vi "THz Time(SR830_ESP300)_Delay_LGS.vi"(1 "ESP300 Axis1":i8=1, 2 "ESP300 Address1":string="1", 4 "Lockin Address":string="12") -> ()   [LabVIEW 2010]
uses:
  <vilib>/Utility/file.llb/Write To Spreadsheet File (DBL).vi
panel:
  out "Boolean 2":bool
  in  "Position 3":sgl=3.0 format="%#.4f"
  in  "Set Position 2":bool
  out "error out":errorcluster
  out "Position 2":dbl[](array[numeric])=[3.0] format="%.6f"
  in  "error in":errorcluster
  out "Running":bool caption="Mercury_GCS_Configuration_Setup.vi is running"
  out "Conn. Axis":string[](array[string])=["1"]
  out "Identification":string="(c)2013 Physik Instrumente(PI) Karlsruhe, C-863.11,0,1.3.0.7"
  in  "SaveFile name":string="t"
  in  "Interdelay (ms)":dbl=10.0
  in  "pre delay(ms)":dbl=100.0
  out "Current deceleration":dbl=100.0
  in  "Acceleration":dbl
  out "Current acceleration":dbl=100.0
  in  "Set Acc":bool
  out "Current Velocity":dbl=25.0
  in  "Delay1 Stage":dbl
  in  "Set Velocity":bool
  in  "Reset Range":bool
  out "Boolean":bool
  out "MinValue":dbl format="%#.3p"
  out "MinPosition":dbl format="%#.3f"
  out "Lock-in Y-Channel":dbl=-8.0036e-11 format="%#.3p"
  out "Lock-in X-Channel":dbl=5.62071e-10 format="%#.3p"
  out "THz Time-domain Signal Wave":cluster{"x-axis":sgl[], "y-axis":dbl[]}(graph)={"x-axis"=[-2.75, -2.745, -2.74, -2.735, -2.73, -2.725, -2.72, -2.715, -2.71, -2.705, -2.7, -2.695, -2.69, -2.685, -2.68, -2.675, -2.67, -2.665, -2.66, -2.655, -2.65, -2.645, -2.64, -2.635, -2.63, -2.625, -2.62, -2.615, -2.61, -2.605, -2.6, -2.595, -2.59, -2.585, -2.58, -2.575, -2.57, -2.565, -2.56, -2.555, -2.55, -2.545, -2.54, -2.535, -2.53, -2.525, -2.52, -2.515, -2.51, -2.505, -2.5, -2.4950001, -2.49, -2.485, -2.48, -2.475, -2.47, -2.465, -2.46, -2.455, -2.45, -2.445, -2.44, -2.435, -2.43, -2.425, -2.42, -2.415, -2.41, -2.405, -2.4, -2.395, -2.39, -2.385, -2.38, -2.375, -2.3700001, -2.365, -2.36, -2.355, -2.35, -2.345, -2.34, -2.335, -2.33, -2.325, -2.32, -2.315, -2.31, -2.305, -2.3, -2.295, -2.29, -2.285, -2.28, -2.275, -2.27, -2.265, -2.26, -2.255, -2.25, -2.2450001, -2.24, -2.235, -2.23, -2.225, -2.22, -2.215, -2.21, -2.205, -2.2, -2.195, -2.19, -2.185, -2.18, -2.175, -2.17, -2.165, -2.16, -2.155, -2.15, -2.145, -2.14, -2.135, -2.13, -2.125, -2.1200001, -2.115, -2.1100001, -2.105, -2.1, -2.095, -2.09, -2.085, -2.08, -2.075, -2.07, -2.065, -2.06, -2.055, -2.05, -2.045, -2.04, -2.035, -2.03, -2.025, -2.02, -2.015, -2.01, -2.005, -2.0, -1.995, -1.99, -1.985, -1.98, -1.975, -1.97, -1.965, -1.96, -1.955, -1.95, -1.945, -1.94, -1.9350001, -1.9300001, -1.9250001, -1.9200001, -1.915, -1.91, -1.905, -1.9, -1.895, -1.89, -1.885, -1.88, -1.875, -1.87, -1.865, -1.86, -1.855, -1.85, -1.845, -1.84, -1.835, -1.83, -1.825, -1.82, -1.815, -1.8100001, -1.8050001, -1.8000001, -1.7950001, -1.79, -1.785, -1.78, -1.775, -1.77, -1.765, -1.76, -1.755, -1.75, -1.745], "y-axis"=array[202 elements]}
  in  "Autosave Directory for Long-term Average Scan":path=path "D:/Soon/140901_delay_test/2_VC_delay_ESP_-2.35/2_ESP_delay"
  out "Phase":cluster{"f0":dbl, "df":dbl, "magnitude":dbl[]}(graph)={"f0"=0.0, "df"=0.14851486070616432, "magnitude"=[3.141592653589793, -1.135986580040852, 2.1022109002271616, -0.606224595657138, 2.920681076611292, 0.21556372083252148, -2.5451476520052716, 0.9923939961615453, -1.7463610341623916, 1.8333042754436455, -0.8359836995409918, 2.75507186449797, 0.09169493821671801, -2.671398777194605, 0.9252867844951119, -1.8804339733205764, 1.635385337194291, -1.1519546083083008, 2.397714684588004, 1.2104854849686713, -2.8637531980944555, 1.949308293908791, 0.7861851325694362, 2.05817428941482, -0.20905665475156449, 2.1403175698295978, 0.5803199632569114, 2.0240075732653433, 2.7198480916992196, 1.4424734657875855, -2.685986408674916, 1.659408491765386, -1.770724027329074, 2.081076418078137, 0.08608209088206076, 2.493628967277787, 1.3416383131006835, 2.776511176774577, 1.7385392296843876, 2.910643788155704, 2.0733616555355256, 2.1476846304355526, 2.3752410087260474, 1.8644630479941513, 2.5623127875118348, 2.148045822962683, 2.289396670128229, 2.4297700200498875, 2.095071647481632, 2.572627457331977, 2.109964594823839, 2.6198261810673187, 2.2914243248471258, 2.3594402988625824, 2.5589534913230425, 1.7745700362271504, 2.954962782799749, 1.86194698187105, -3.1249566392866623, 2.2303719482942626, 2.6892266936683993, 2.5935042746540447, 2.41043968808954, 2.6541419887600273, 2.683074815417406, 2.1668243385246915, -3.070776678111956, 2.2892022436016632, -2.135166602508625, 2.7313396286767393, 1.2942375262133383, -2.98549486935882, 2.211769682179136, -1.9765629636412416, 2.8315046162560114, 0.8982661941803926, 3.0979638891430006, 1.3338431160230941, 2.9572589462558923, 0.4208158598849399, -3.084879211462056, 1.1546365000649987, -2.426896356838734, 2.1224318208935746, -1.0822400276671367, -3.138191445873515, 1.3677675484659175, -2.1384004116313586, 2.2666526927596524, -0.9626777899091671, 2.9711856946896824, 0.5728247348162799, -2.816675001259512, 1.473325365303859, -2.6794056673427953, 1.5349065678241745, -2.6858532380239843, 1.534598210049353, -2.4469347300537185, 2.0442041388150147, -2.311182814513963]}
  out "elapsed time":string=" 0 h  16 m  48 s"
  in  "OK Button":bool
  out "Data Type":string="outp ? 1"
  in  "Enum":enum16{"X", "Y", "Abs"}(ring)
  out "MaxValue":dbl format="%#.3p"
  out "MaxPosition":dbl format="%#.3f"
  in  "Position":sgl format="%#.4f"
  in  "Find Max":bool
  in  "Set Position":bool
  in  "Save Data":bool
  in  "SCAN":bool
  in  "Exit Program":bool
  out "Amplitude":cluster{"f0":dbl, "df":dbl, "magnitude":dbl[]}(graph)={"f0"=0.0, "df"=0.14851486070616432, "magnitude"=[2.6915991854888386e-11, 8.375656748039542e-10, 2.235834721082622e-09, 3.4157684600132285e-09, 4.2435755658762315e-09, 4.472539329076285e-09, 4.2347337941880014e-09, 3.6229569047721997e-09, 2.7975925998611847e-09, 2.0909687588148054e-09, 1.4776684583256283e-09, 1.0684148893892852e-09, 7.434640997068466e-10, 5.034295148742816e-10, 3.3364314234066716e-10, 1.9577697939408548e-10, 1.2523927442263667e-10, 4.429210924914903e-11, 2.573647079693204e-11, 1.4182414959459453e-11, 2.7755861329404263e-12, 1.4087176698727024e-11, 1.3906256401648906e-12, 1.3855617151926235e-11, 2.3183905698719347e-12, 1.3260260840826552e-11, 1.6764421372823549e-12, 9.240136905598061e-12, 4.112473401393782e-12, 9.698672089635608e-12, 6.399880474780534e-12, 1.3297238354970657e-11, 4.270910531055341e-12, 1.194277964154244e-11, 2.0143741595524134e-12, 8.19663059000381e-12, 4.499163612930761e-12, 4.984976956409621e-12, 5.930135725317639e-12, 2.6529048225466805e-12, 6.413329122555876e-12, 1.5875211615976485e-12, 5.603892306521492e-12, 3.0822718239556447e-12, 3.773490804705028e-12, 4.266071720358043e-12, 2.7269286375688967e-12, 4.04702550108293e-12, 3.1385561228088536e-12, 3.5820473163129804e-12, 3.4584571573909894e-12, 2.8260585036815302e-12, 3.954420907012932e-12, 2.109422403518565e-12, 4.405123782627864e-12, 2.328141166049999e-12, 4.110618048699576e-12, 3.7699178777659875e-12, 2.75243386150393e-12, 4.1423186986189514e-12, 1.889383468271808e-12, 3.468042829240754e-12, 2.7069840219363736e-12, 2.355134561389352e-12, 3.3764264273860032e-12, 2.5890110570824253e-12, 2.645733242043269e-12, 4.509912096670506e-12, 7.24673781011345e-13, 5.531658054842724e-12, 1.7743067719520671e-12, 3.936201982796357e-12, 4.271899404256137e-12, 8.217749918070464e-13, 5.699197262594634e-12, 1.5430271083565579e-12, 5.25759708946632e-12, 1.449496509764676e-12, 5.3347687277906044e-12, 1.804360465622194e-12, 6.9752988572067005e-12, 4.2197168647319695e-12, 5.704160353607782e-12, 5.79769144265315e-12, 2.0168312984405185e-12, 6.483488385921406e-12, 4.16443233788095e-12, 5.524003351010582e-12, 6.9219189903466406e-12, 3.2560936701576393e-12, 7.2038923234186815e-12, 2.643003207182121e-12, 6.1557127448571425e-12, 3.009475442598e-12, 5.064751562703159e-12, 2.590926363995777e-12, 5.492940598962602e-12, 3.266879593571407e-12, 5.207284837307166e-12, 3.5754755911677846e-12, 2.6128905192061403e-12]}
  in  "Short term \nAverage#":i8=2
  out "Numeric 2":i8=15
  in  "Long term Average#":i8=16
  in  "Step":sgl=0.005 min=0 max=10000 format="%.3f"
  in  "End Postion":sgl=-1.75 min=-400 max=400 format="%#.3f"
  in  "Start Position":sgl=-2.75 min=-400 max=400 format="%#.3f"
  # "This Program Run First (1) and then Run the Approach Program (2)"
  # "THz Experiment"
  # "``"
  # "Auto-offset"
  # "Input Data"
  # "Delay Line (ESP300)"
  # "Point Avg"
  # "Long Avg"
  # "Turn Number"
  # "mm"
  # "mm"
  # "MAX"
  # "MIN"
  # "other step\nposition"
  # "stage \nposition"
  # "stage \nposition"
  # "value"
  # "value"
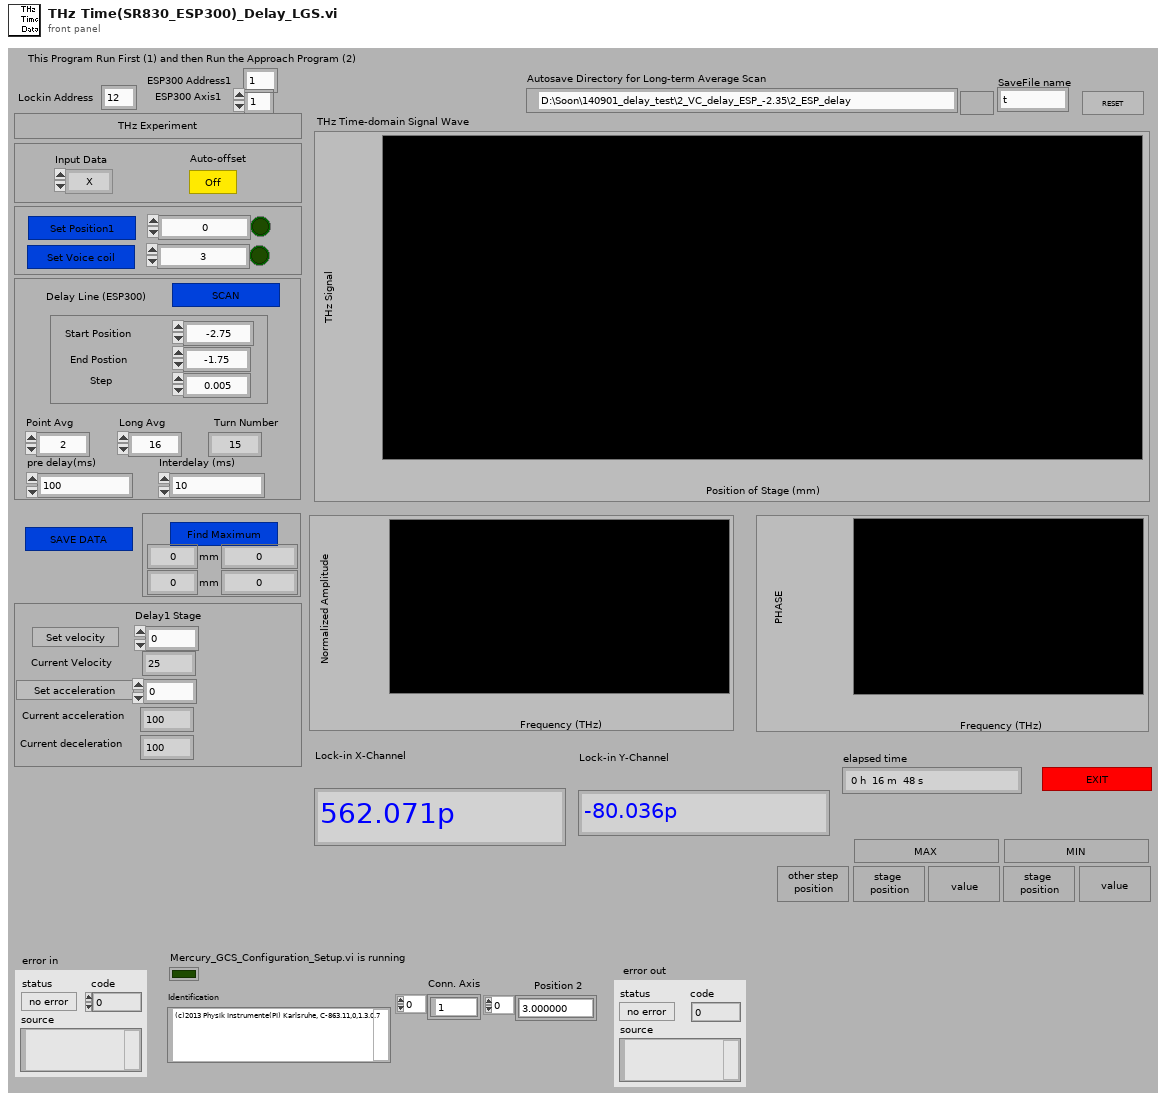
[diagram p1: front panel]
types:
  T1 = cluster{"System no.":i32, "error out":errorcluster}
  T2 = cluster{"Step Number":i32, "Step":sgl, "Start Position":sgl, "Time-out":i32, "Lockin Address":string, "Short term \nAverage#":i8, i32, "ESP300 Axis1":i8, "Value":string, "pre delay(ms)":dbl, "Interdelay (ms)":dbl, "Autosave Directory for Long-term Average Scan":path}
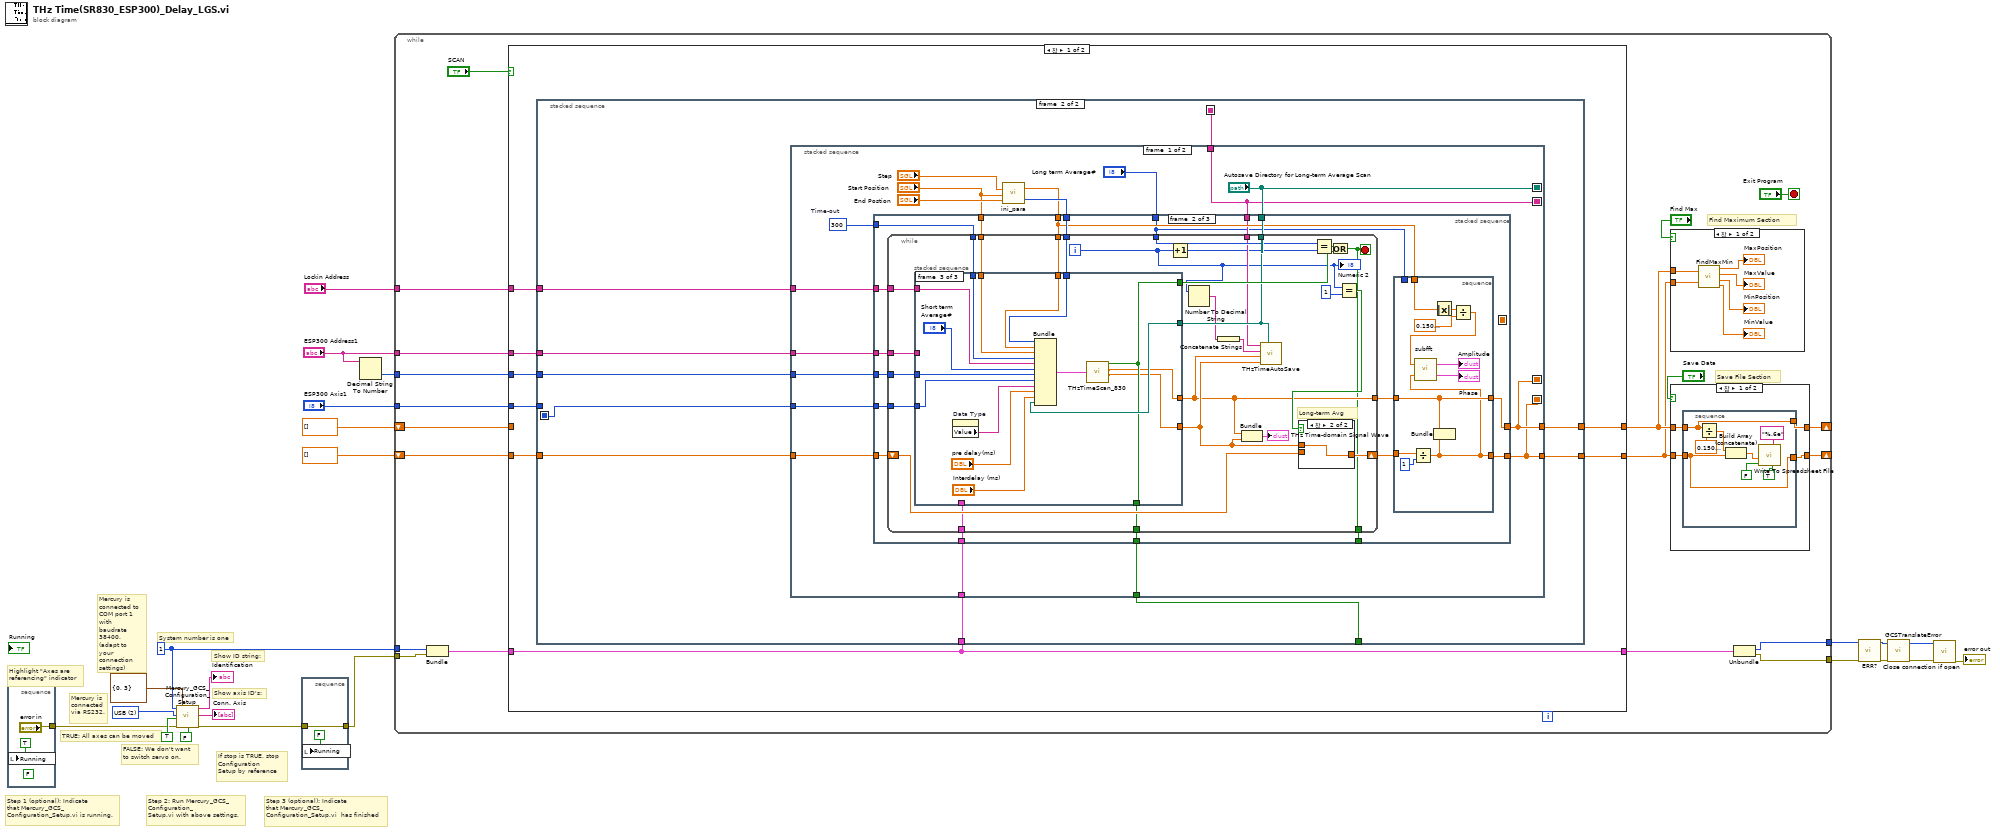
[diagram p0: block diagram]
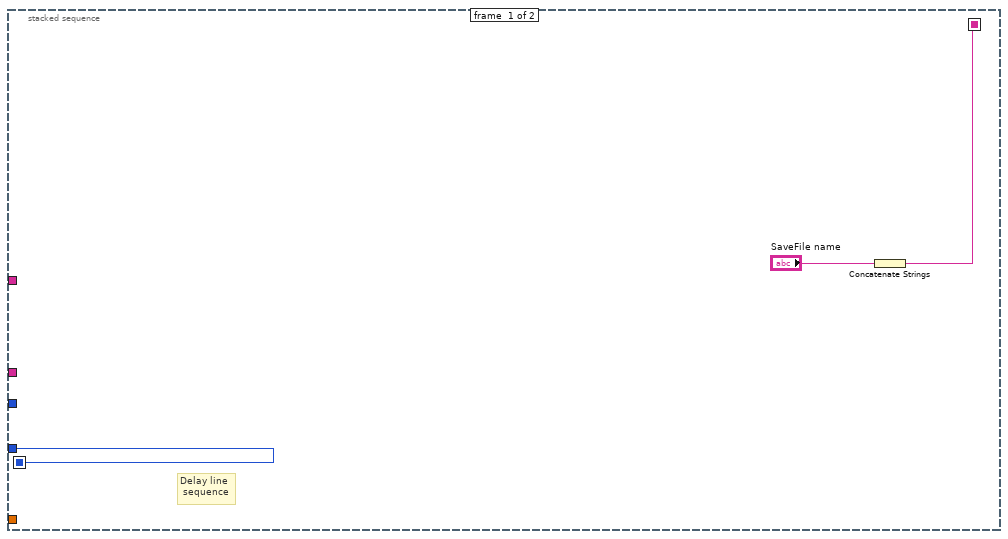
[diagram p4: hidden frame]
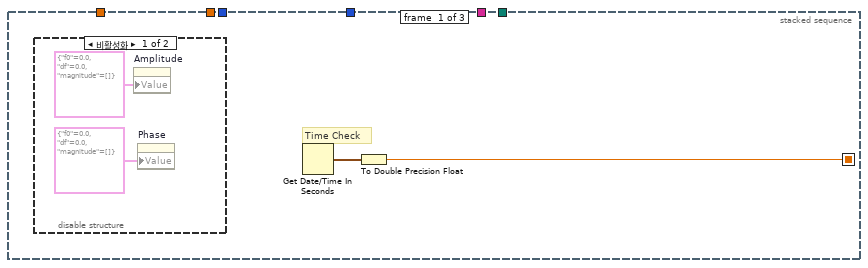
[diagram p5: hidden frame]
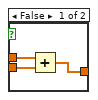
[diagram p7: hidden frame]
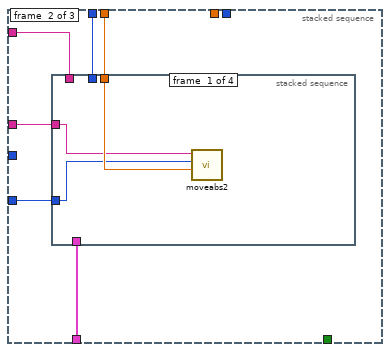
[diagram p9: hidden frame]
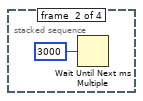
[diagram p10: hidden frame]
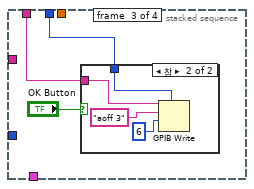
[diagram p11: hidden frame]
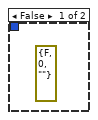
[diagram p12: hidden frame]
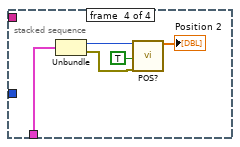
[diagram p13: hidden frame]
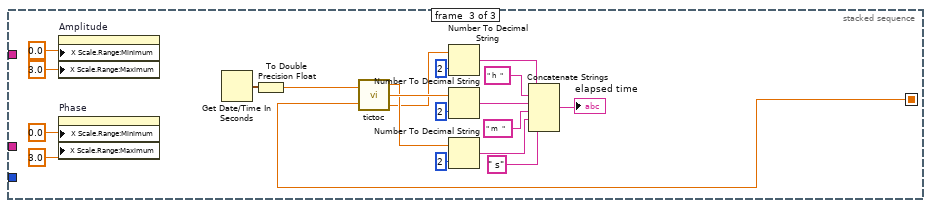
[diagram p14: hidden frame]
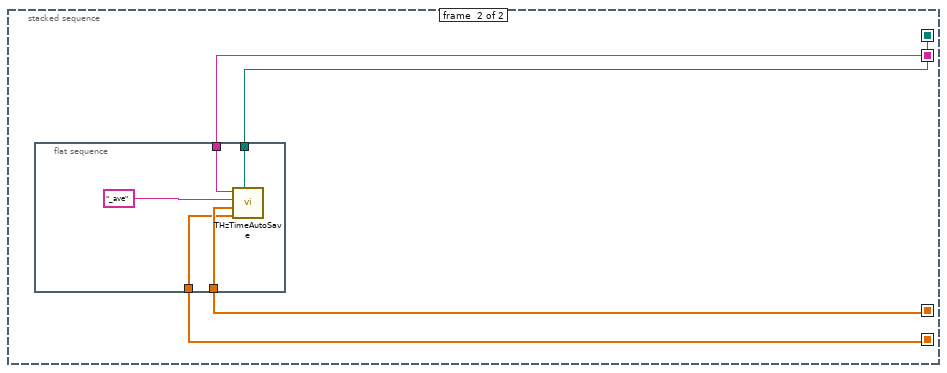
[diagram p15: hidden frame]
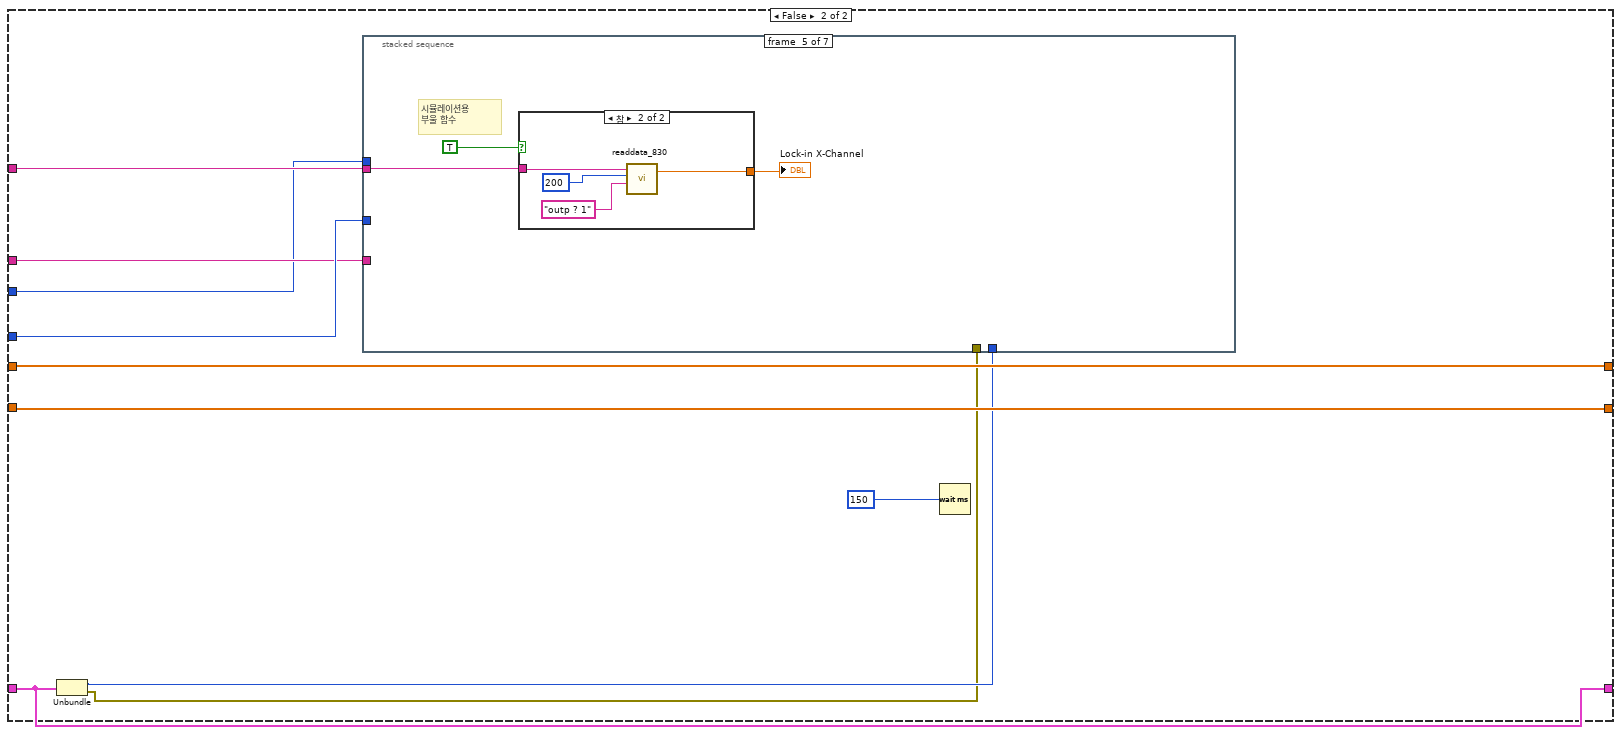
[diagram p16: hidden frame]
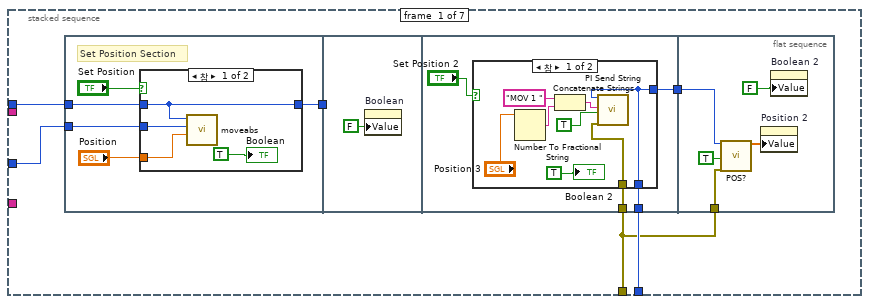
[diagram p17: hidden frame]
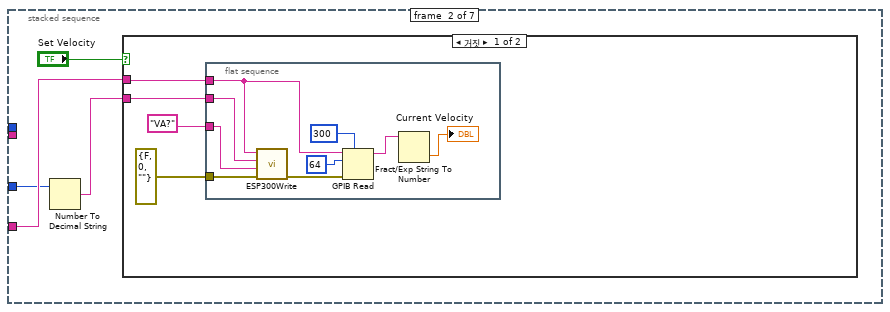
[diagram p20: hidden frame]
diagram:
  w8 = u16 2 items=["RS232", "RS232 DaisyChain", "USB", "USB_DaisyChain"] ("Interface")
  w7 = 1 ("System no.")
  # "Mercury is\nconnected\nvia RS232."
  # "If stop is TRUE, stop \nConfiguration\nSetup by reference"
  # "Mercury is\nconnected to\nCOM port 1\nwith baudrate\n38400.\n(adapt to your\nconnection\nsettings)"
  # "Step 3 (optional): Indicate\nthat Mercury_GCS_\nConfiguration_Setup.vi  has finished"
  # "Step 2: Run Mercury_GCS_\nConfiguration_\nSetup.vi with above settings."
  # "Step 1 (optional): Indicate\nthat Mercury_GCS_\nConfiguration_Setup.vi is running."
  # "Highlight \"Axes are\nreferencing\" indicator"
  # "Show axis ID's:"
  # "Show ID string:"
  # "FALSE: We don't want\nto switch servo on."
  # "TRUE: All axes can be moved"
  # "System number is one"
  n1 = stacked-sequence {
    tunnel: ["error in"] -> w11
    frame #0 {
      (unwired) FALSE ("stop")
      n2 = local write "Running"(TRUE ("Running")) -> ()
    }
  }
  n3 = call "Mercury_GCS_Configuration_Setup.vi"("System no."=w7, "Interface"=w8, "All axes?"=TRUE, "error in"=w11, "RS232 settings"=cluster{"RS232 Portnumber":i32, "Baudrate":u16} {"RS232 Portnumber"=0, "Baudrate"=3}, "Switch servo on?"=FALSE ("Use dialog to define\nconnected stages?")) -> ("Identification"=→"Identification":string, "Conn. \nAxes"=→"Conn. Axis":string[], "error out"=w12:errorcluster)  [unwired: 7 in, 4 out]
  n4 = stacked-sequence {
    tunnel: w12 -> [w25]
    tunnel: [w25] -> w6
    frame #0 {
      n5 = local write "Running"(FALSE ("Running")) -> ()
    }
  }
  n6 = Decimal String To Number(string="ESP300 Address1") -> (number=w16:i32)  [unwired: 2 in, 1 out]
  n7 = while {
    tunnel: "ESP300 Axis1" -> [w41]
    tunnel: "Lockin Address" -> [w33]
    shift-right: [w38] -> _
    shift-left: sgl[] [] -> [w40]
    shift-right: [w37] -> _
    shift-left: dbl[] [] -> [w39]
    tunnel: "ESP300 Address1" -> [w34]
    tunnel: w16 -> [w32]
    tunnel: w7 -> [w31]
    tunnel: w6 -> [w30]
    tunnel: [w27] -> w2
    tunnel: [w26] -> w1
    stop <- "Exit Program" stop-if-true
    # "Save File Section"
    # "Find Maximum Section"
    n8 = Bundle("System no."=w31, "error out"=w30) -> (w29:T1)  [unwired: 1 in]
    n9 = case shown="참" "SCAN" {
      tunnel: w41 -> [w73 w245]
      tunnel: [w72 w242] -> w36
      tunnel: [w71 w241] -> w35
      tunnel: w40 -> [_ w242]
      tunnel: w39 -> [w70 w241]
      tunnel: w34 -> [w69 w243]
      tunnel: w33 -> [w68 w240]
      tunnel: w32 -> [w67 w239]
      tunnel: w29 -> [w66 w236]
      tunnel: [w66 w236] -> w28
      frame True {
        n10 = stacked-sequence {
          seq-local: [w76 _] -> [_ w79]
          seq-local: [w74 _] -> [_ w80]
          tunnel: w73 -> [w76 _]
          tunnel: [_ w86] -> w72
          tunnel: [_ w85] -> w71
          tunnel: w70 -> [_ w84]
          tunnel: w69 -> [_ w83]
          tunnel: w68 -> [_ w82]
          tunnel: w67 -> [_ w81]
          tunnel: [_ w77] -> _
          tunnel: w66 -> [_ w78]
          frame #0 {
            # "Delay line\n sequence"
            n11 = Concatenate Strings("SaveFile name") -> (w74:string)
          }
          frame #1 {
            n12 = stacked-sequence {
              seq-local: [w94 _] -> [_ w228]
              seq-local: [w93 _] -> [_ w227]
              seq-local: ["Autosave Directory for Long-term Average Scan" _] -> [_ w229]
              seq-local: [w89 _] -> [_ w230]
              tunnel: w79 -> [w104 _]
              tunnel: [w94 _] -> w86
              tunnel: [w93 _] -> w85
              tunnel: w84 -> [w97 _]
              tunnel: w83 -> [w96 _]
              tunnel: [w95 _] -> w77
              tunnel: w82 -> [w91 _]
              tunnel: w81 -> [w90 _]
              tunnel: w80 -> [w89 _]
              tunnel: w78 -> [w87 _]
              frame #0 {
                w103 = 300  # Time-out
                n13 = call "ini_para.vi"("End Position"="End Postion", "Start Position"="Start Position", "Step"="Step") -> ("Step Number"=w100:i32, "Step"=w99:sgl)
                n14 = stacked-sequence {
                  seq-local: [w105 _ _] -> [_ _ w207]
                  tunnel: w103 -> [_ w127 _]
                  tunnel: "Long term Average#" -> [_ w110 _]
                  tunnel: w104 -> [_ w126 _]
                  tunnel: w100 -> [_ w124 _]
                  tunnel: w99 -> [_ w122 _]
                  tunnel: "Start Position" -> [_ w125 _]
                  tunnel: "Autosave Directory for Long-term Average Scan" -> [_ w123 _]
                  tunnel: [_ w113 _] -> w94
                  tunnel: [_ w121 _] -> w93
                  tunnel: w97 -> [_ w119 _]
                  tunnel: w96 -> [_ w120 _]
                  tunnel: w89 -> [_ w118 _]
                  tunnel: [_ w117 _] -> w95
                  tunnel: w91 -> [_ w116 _]
                  tunnel: w90 -> [_ w115 _]
                  tunnel: [_ w111 _] -> _
                  tunnel: w87 -> [_ w109 _]
                  frame #0 {
                    # "Time Check"
                    n15 = disable-structure shown="비활성화" {
                      frame Disabled {
                        n16 = property on="Amplitude" class="WFGraph (엄격한)"("Value"=cluster{"f0":dbl, "df":dbl, "magnitude":dbl[]} {"f0"=0.0, "df"=0.0, "magnitude"=[]} ("Spectrum")) -> ()  [unwired: 2 in, 2 out]
                        n17 = property on="Phase" class="WFGraph (엄격한)"("Value"=cluster{"f0":dbl, "df":dbl, "magnitude":dbl[]} {"f0"=0.0, "df"=0.0, "magnitude"=[]} ("Spectrum")) -> ()  [unwired: 2 in, 2 out]
                      }
                      frame Enabled {
                      }
                    }
                    n18 = Get Date/Time In Seconds() -> (seconds since 1Jan1904=w106:timestamp)
                    n19 = To Double Precision Float(number=w106) -> (double precision float=w105:dbl)
                  }
                  frame #1 {
                    n20 = while {
                      tunnel: w110 -> [w163]
                      tunnel: w127 -> [w164]
                      tunnel: w126 -> [w160]
                      tunnel: w125 -> [w159]
                      tunnel: w122 -> [w158]
                      tunnel: w124 -> [w157]
                      tunnel: w123 -> [w152]
                      shift-right: [w142] -> w112
                      shift-left: w119 -> [w155]
                      tunnel: [w145] -> w114
                      tunnel: w120 -> [w154]
                      tunnel: w118 -> [w151]
                      tunnel: [w153] -> w117
                      tunnel: w116 -> [w148]
                      tunnel: w115 -> [w147]
                      tunnel: [w141] -> w111
                      tunnel: w109 -> [w138]
                      i -> [w139]
                      stop <- w141 stop-if-true
                      # "Long-term Avg"
                      n21 = stacked-sequence {
                        tunnel: w164 -> [_ w174 w205]
                        tunnel: [_ _ w193] -> w161
                        tunnel: w160 -> [_ w173 w196]
                        tunnel: w159 -> [_ w172 w197]
                        tunnel: w158 -> [_ _ w198]
                        tunnel: w157 -> [_ _ w206]
                        tunnel: [_ _ w192] -> w145
                        tunnel: [_ _ w191] -> w149
                        tunnel: w154 -> [_ w171 _]
                        tunnel: w152 -> [_ _ w200]
                        tunnel: [_ _ w193] -> w153
                        tunnel: w148 -> [_ w170 w199]
                        tunnel: w147 -> [_ _ w195]
                        tunnel: w138 -> [_ w169 _]
                        frame #0 {
                        }
                        frame #1 {
                          n22 = stacked-sequence {
                            tunnel: w174 -> [_ _ w180 _]
                            tunnel: w173 -> [w175 _ _ _]
                            tunnel: w172 -> [w177 _ _ _]
                            tunnel: w171 -> [w176 _ _ _]
                            tunnel: w170 -> [_ _ w179 _]
                            tunnel: w169 -> [_ _ _ w188]
                            frame #0 {
                              n23 = call "moveabs2.vi"("SetPosition"=w177, "EXP300 Axis"=w175, "THz Image\nESP Address"=w176) -> ()  [unwired: 1 in, 1 out]
                            }
                            frame #1 {
                              n24 = Wait Until Next ms Multiple(millisecond multiple=3000) -> ()  [unwired: 1 out]
                            }
                            frame #2 {
                              n25 = case shown="참" "OK Button" {
                                tunnel: w180 -> [_ w184]
                                tunnel: w179 -> [_ w182]
                                frame False {
                                (unwired) errorcluster {"status"=FALSE, "code"=0, "source"=""} ("error in")
                                }
                                frame True {
                                n26 = GPIB Write(0:w182, 1:"aoff 3" ("data"), 2:i16 6 ("mode (0)"), 4:w184) -> ()  [unwired: 1 in, 2 out]
                                }
                              }
                            }
                            frame #3 {
                              n27 = Unbundle(w188) -> ("System no."=w187:i32, "error out"=w186:errorcluster)
                              n28 = call "POS?.vi"("System no."=w187, "All axes?"=TRUE, "error in"=w186) -> ("Position"=→"Position 2":dbl[])  [unwired: 15 in, 1 out]
                            }
                          }
                        }
                        frame #2 {
                          n29 = property on="Data Type" class="Str"() -> ("Value"=w203:string)  [unwired: 2 in, 2 out]
                          n30 = Bundle("Step Number"=w206, "Step"=w198, "Start Position"=w197, "Time-out"=w205, "Lockin Address"=w199, "Short term \nAverage#"="Short term \nAverage#", w195, "ESP300 Axis1"=w196, "Value"=w203, "pre delay(ms)"="pre delay(ms)", "Interdelay (ms)"="Interdelay (ms)", "Autosave Directory for Long-term Average Scan"=w200) -> (w194:T2)  [unwired: 1 in]
                          n31 = call "THzTimeScan_830.vi"("input"=w194) -> ("loop stop"=w193:bool, "x-axis"=w192:sgl[], "y-axis"=w191:dbl[])  [unwired: 1 in]
                        }
                      }
                      n32 = Increment(x=w139) -> (x+1=w143:i32)
                      n33 = Number To Decimal String(number=w139) -> (decimal integer string=w140:string)  [unwired: 1 in]
                      n34 = Concatenate Strings(w140) -> (w150:string)
                      n35 = Bundle("x-axis"=w145, "y-axis"=w149) -> (→"THz Time-domain Signal Wave":cluster{"x-axis":sgl[], "y-axis":dbl[]})  [unwired: 1 in]
                      n36 = call "THzTimeAutoSave.vi"("Autosave Directory for Long-term Average Scan"=w152, "y-axis"=w149, "x-axis"=w145, "String"=w150, "SaveFile name"=w151) -> ()  [unwired: 5 in]
                      n37 = Equal?(x=w163, y=w143) -> (x = y?=w162:bool)
                      n38 = Or(x=w162, y=w161) -> (x .or. y?=w141:bool)
                      n39 = Equal?(x=w139, y=1) -> (x = y?=w146:bool)
                      n40 = case shown="참" w146 {
                        tunnel: w155 -> [w166 _]
                        tunnel: w149 -> [w167 w168]
                        tunnel: [w165 w168] -> w142
                        frame False {
                          n41 = Add(x=w167, y=w166) -> (x+y=w165:dbl[])
                        }
                        frame True {
                        }
                      }
                      "Numeric 2" <- w139
                    }
                    n42 = stacked-sequence {
                      tunnel: w122 -> [w133]
                      tunnel: w114 -> [w130]
                      tunnel: w112 -> [w131]
                      tunnel: [w129] -> w121
                      tunnel: w110 -> [_]
                      tunnel: [w130] -> w113
                      frame #0 {
                        n43 = Divide(x=w131, y=1) -> (x/y=w129:dbl[])
                        n44 = Absolute Value(x=w133) -> (abs(x)=w134:sgl)
                        n45 = Bundle("x-axis"=w130, w129) -> ()  [unwired: 1 in, 1 out]
                        n46 = Divide(x=w134, y=sgl 0.15) -> (x/y=w132:sgl)
                        n47 = call "subfft.vi"("y-signal"=w129, "time step"=w132) -> ("Phase"=→"Phase":cluster{"f0":dbl, "df":dbl, "real part":dbl[]}, "Amplitude"=→"Amplitude":cluster{"f0":dbl, "df":dbl, "real part":dbl[]})
                      }
                    }
                  }
                  frame #2 {
                    n48 = property on="Amplitude" class="WFGraph (엄격한)"("X Scale.Range:Minimum"=0.0 ("X Scale.Range:Maximum"), "X Scale.Range:Maximum"=3.0) -> ()  [unwired: 2 in, 2 out]
                    n49 = property on="Phase" class="WFGraph (엄격한)"("X Scale.Range:Minimum"=0.0, "X Scale.Range:Maximum"=3.0) -> ()  [unwired: 2 in, 2 out]
                    n50 = Get Date/Time In Seconds() -> (seconds since 1Jan1904=w212:timestamp)
                    n51 = To Double Precision Float(number=w212) -> (double precision float=w211:dbl)
                    n52 = call "tictoc.vi"("Value"=w211, "Value 2"=w207) -> ("sec"=w209:dbl, "min"=w210:dbl, "hour"=w208:dbl)
                    n53 = Number To Decimal String(number=w208, width (-)=i16 2) -> (decimal integer string=w217:string)
                    n54 = Number To Decimal String(number=w210, width (-)=i16 2) -> (decimal integer string=w223:string)
                    n55 = Number To Decimal String(number=w209, width (-)=i16 2) -> (decimal integer string=w222:string)
                    n56 = Concatenate Strings(w217, " h  " ("Substring"), w223, " m  " ("Substring"), w222, " s" ("Substring")) -> (→"elapsed time":string)
                  }
                }
              }
              frame #1 {
                n57 = flat-sequence {
                  tunnel: w229 -> [w235]
                  tunnel: w230 -> [w234]
                  tunnel: w228 -> [w233]
                  tunnel: w227 -> [w232]
                  frame #0 {
                    n58 = call "THzTimeAutoSave.vi"("Autosave Directory for Long-term Average Scan"=w235, "y-axis"=w232, "x-axis"=w233, "String"="_ave" ("string"), "SaveFile name"=w234) -> ()  [unwired: 5 in]
                  }
                }
              }
            }
          }
        }
      }
      frame False {
        n59 = Unbundle(w236) -> ("System no."=w238:i32, "error out"=w237:errorcluster)
        n60 = stacked-sequence {
          tunnel: w245 -> [w251 w282 w311 _ _ _ _]
          tunnel: w243 -> [_ w283 w312 _ _ _ _]
          tunnel: w240 -> [_ _ _ _ w369 w378 _]
          tunnel: w239 -> [w250 _ _ _ _ _ _]
          tunnel: w238 -> [w248 _ _ _ _ _ _]
          tunnel: w237 -> [w246 _ _ _ _ _ _]
          frame #0 {
            n61 = flat-sequence {
              tunnel: w251 -> [w256]
              tunnel: w250 -> [w253]
              tunnel: [w252] -> w249
              tunnel: w249 -> [_]
              tunnel: w248 -> [w265]
              tunnel: w246 -> [w264]
              tunnel: [w263] -> w247
              tunnel: w247 -> [w278]
              tunnel: w246 -> [w277]
              frame #0 {
                # "Set Position Section"
                n62 = case shown="참" "Set Position" {
                  tunnel: "Position" -> [w260 _]
                  tunnel: w256 -> [w259 _]
                  tunnel: w253 -> [w257 w261]
                  tunnel: [w257 w261] -> w252
                  frame True {
                    n63 = call "moveabs.vi"("SetPosition"=w260, "EXP300 -3A Axis"=w259, "ESP300 -3A Add."=w257) -> ()  [unwired: 2 in]
                    "Boolean" <- TRUE
                  }
                  frame False {
                  }
                }
              }
              frame #1 {
                n64 = property on="Boolean" class="Bool (엄격한)"("Value"=FALSE ("Boolean")) -> ()  [unwired: 2 in, 2 out]
              }
              frame #2 {
                n65 = case shown="참" "Set Position 2" {
                  tunnel: w265 -> [w267 w275]
                  tunnel: w264 -> [w268 _]
                  tunnel: [w267 w275] -> w263
                  frame True {
                    n66 = Number To Fractional String(number="Position 3") -> (F-format string=w270:string)  [unwired: 3 in]
                    n67 = Concatenate Strings("MOV 1 ", w270) -> (w273:string)
                    n68 = call "PI Send String.vi"("System no."=w267, "String to send"=w273, "Attach termination char.?"=TRUE ("Attach Linefeed?"), "error in"=w268) -> ()  [unwired: 15 in, 1 out]
                    "Boolean 2" <- TRUE
                  }
                  frame False {
                  }
                }
              }
              frame #3 {
                n69 = call "POS?.vi"("System no."=w278, "All axes?"=TRUE, "error in"=w277) -> ("Position"=w280:dbl[])  [unwired: 15 in, 1 out]
                n70 = property on="Position 2" class="Arr (엄격한)"("Value"=w280) -> ()  [unwired: 2 in, 2 out]
                n71 = property on="Boolean 2" class="Bool (엄격한)"("Value"=FALSE ("Boolean")) -> ()  [unwired: 2 in, 2 out]
              }
            }
          }
          frame #1 {
            n72 = Number To Decimal String(number=w282) -> (decimal integer string=w281:string)  [unwired: 1 in]
            n73 = case shown="거짓" "Set Velocity" {
              tunnel: w283 -> [w285 w301]
              tunnel: w281 -> [w288 w302]
              frame False {
                n74 = flat-sequence {
                  tunnel: w288 -> [w297]
                  tunnel: errorcluster {"status"=FALSE, "code"=0, "source"=""} ("error in (no error)") -> [w290]
                  tunnel: "VA?" ("Command") -> [w291]
                  tunnel: w285 -> [w289]
                  frame #0 {
                    n75 = call "ESP300Write.vi"("error in (no error)"=w290, "Command"=w291, "ESP300 Axis"=w297, "ESP300 Address"=w289) -> ("error out"=w292:errorcluster)  [unwired: 3 in]
                    n76 = GPIB Read(0:w289, 1:64 ("byte count"), 3:w292, 4:300 ("timeout ms (488.2 global)")) -> (5:w296:string)  [unwired: 1 in, 2 out]
                    n77 = Fract/Exp String To Number(string=w296) -> (number=→"Current Velocity":dbl)  [unwired: 3 in, 1 out]
                  }
                }
              }
              frame True {
                n78 = flat-sequence {
                  tunnel: w302 -> [w310]
                  tunnel: w301 -> [w305]
                  tunnel: [w305] -> w300
                  tunnel: errorcluster {"status"=FALSE, "code"=0, "source"=""} ("error in (no error)") -> [w304]
                  tunnel: [w303] -> w298
                  tunnel: w300 -> [_]
                  tunnel: w298 -> [_]
                  frame #0 {
                    n79 = Number To Fractional String(number="Delay1 Stage") -> (F-format string=w308:string)  [unwired: 3 in]
                    n80 = Concatenate Strings("VA" ("string"), w308) -> (w306:string)
                    n81 = call "ESP300Write.vi"("error in (no error)"=w304, "Command"=w306, "ESP300 Axis"=w310, "ESP300 Address"=w305) -> ("error out"=w303:errorcluster)  [unwired: 3 in]
                  }
                  frame #1 {
                  }
                }
              }
            }
          }
          frame #2 {
            n82 = Number To Decimal String(number=w311) -> (decimal integer string=w313:string)  [unwired: 1 in]
            n83 = case shown="참" "Set Acc" {
              tunnel: w312 -> [w315 w340]
              tunnel: w313 -> [w316 w341]
              frame False {
                n84 = stacked-sequence {
                  tunnel: w316 -> [w318 w328]
                  tunnel: w315 -> [w317 w329]
                  frame #0 {
                    n85 = flat-sequence {
                      tunnel: w318 -> [w327]
                      tunnel: w317 -> [w320]
                      frame #0 {
                        n86 = call "ESP300Write.vi"("error in (no error)"=errorcluster {"status"=FALSE, "code"=0, "source"=""}, "Command"="AC?", "ESP300 Axis"=w327, "ESP300 Address"=w320) -> ("error out"=w321:errorcluster)  [unwired: 3 in]
                        n87 = GPIB Read(0:w320, 1:64 ("byte count"), 3:w321, 4:300 ("timeout ms (488.2 global)")) -> (5:w325:string)  [unwired: 1 in, 2 out]
                        n88 = Fract/Exp String To Number(string=w325) -> (number=→"Current acceleration":dbl)  [unwired: 3 in, 1 out]
                      }
                    }
                  }
                  frame #1 {
                    n89 = flat-sequence {
                      tunnel: w328 -> [w338]
                      tunnel: w329 -> [w332]
                      frame #0 {
                        n90 = call "ESP300Write.vi"("error in (no error)"=errorcluster {"status"=FALSE, "code"=0, "source"=""}, "Command"="AG?", "ESP300 Axis"=w338, "ESP300 Address"=w332) -> ("error out"=w333:errorcluster)  [unwired: 3 in]
                        n91 = GPIB Read(0:w332, 1:64 ("byte count"), 3:w333, 4:300 ("timeout ms (488.2 global)")) -> (5:w336:string)  [unwired: 1 in, 2 out]
                        n92 = Fract/Exp String To Number(string=w336) -> (number=→"Current deceleration":dbl)  [unwired: 3 in, 1 out]
                      }
                    }
                  }
                }
              }
              frame True {
                n93 = stacked-sequence {
                  seq-local: [w343 _] -> [_ w354]
                  tunnel: w340 -> [w345 w356]
                  tunnel: w341 -> [w344 w355]
                  tunnel: errorcluster {"status"=FALSE, "code"=0, "source"=""} ("error in (no error)") -> [w342 w353]
                  frame #0 {
                    n94 = flat-sequence {
                      tunnel: w344 -> [w352]
                      tunnel: w345 -> [w348]
                      tunnel: ["Acceleration"] -> w343
                      tunnel: w342 -> [w346]
                      frame #0 {
                        n95 = Number To Fractional String(number="Acceleration") -> (F-format string=w351:string)  [unwired: 3 in]
                        n96 = Concatenate Strings("AC" ("string"), w351) -> (w349:string)
                        n97 = call "ESP300Write.vi"("error in (no error)"=w346, "Command"=w349, "ESP300 Axis"=w352, "ESP300 Address"=w348) -> ()  [unwired: 3 in, 1 out]
                      }
                    }
                  }
                  frame #1 {
                    n98 = flat-sequence {
                      tunnel: w355 -> [w363]
                      tunnel: w356 -> [w359]
                      tunnel: w354 -> [w358]
                      tunnel: w353 -> [w357]
                      frame #0 {
                        n99 = Number To Fractional String(number=w358) -> (F-format string=w362:string)  [unwired: 3 in]
                        n100 = Concatenate Strings("AG" ("string"), w362) -> (w360:string)
                        n101 = call "ESP300Write.vi"("error in (no error)"=w357, "Command"=w360, "ESP300 Axis"=w363, "ESP300 Address"=w359) -> ()  [unwired: 3 in, 1 out]
                      }
                    }
                  }
                }
              }
            }
          }
          frame #3 {
            # "Data Type Select"
            n102 = case shown="\"X\", 기본" "Enum" {
              tunnel: ["outp ? 1" "outp ? 2" "outp ? 3"] -> w365
              frame "X", Default {
              }
              frame "Y" {
              }
              frame "Abs" {
              }
            }
            "Data Type" <- w365
          }
          frame #4 {
            # "시뮬레이션용\n부울 함수"
            n103 = case shown="참" TRUE {
              tunnel: [w372 w374] -> w371
              tunnel: w369 -> [_ w373]
              frame False {
                n104 = Random Number (0-1)() -> (number: 0 to 1=w372:dbl)
              }
              frame True {
                n105 = call "readdata_830.vi"("Command"="outp ? 1", "timeout"=200, "Lockin Address"=w373) -> ("Data"=w374:dbl)  [unwired: 1 in, 1 out]
              }
            }
            "Lock-in X-Channel" <- w371
          }
          frame #5 {
            n106 = case shown="참" TRUE {
              tunnel: w378 -> [_ w382]
              tunnel: [w380 w381] -> w377
              frame False {
                n107 = Random Number (0-1)() -> (number: 0 to 1=w380:dbl)
              }
              frame True {
                n108 = call "readdata_830.vi"("Command"="outp ? 2", "timeout"=200, "Lockin Address"=w382) -> ("Data"=w381:dbl)  [unwired: 1 in, 1 out]
              }
            }
            "Lock-in Y-Channel" <- w377
          }
          frame #6 {
            n109 = case shown="거짓" "Reset Range" {
              frame False {
              }
              frame True {
                n110 = property on="Start Position" class="DigNum (엄격한)"() -> ("Value"=w387:sgl)  [unwired: 2 in, 2 out]
                n111 = property on="End Postion" class="DigNum (엄격한)"() -> ("Value"=w386:sgl)  [unwired: 2 in, 2 out]
                n112 = property on="THz Time-domain Signal Wave" class="XYGraph (엄격한)"("X Scale.Range:Minimum"=w387, "X Scale.Range:Maximum"=w386) -> ()  [unwired: 2 in, 2 out]
              }
            }
          }
        }
        n113 = Wait (ms)(milliseconds to wait=u32 150) -> ()  [unwired: 1 out]
      }
    }
    n114 = case shown="참" "Find Max" {
      tunnel: w36 -> [w65 _]
      tunnel: w35 -> [w64 _]
      frame True {
        n115 = call "FindMaxMin.vi"("x-axis"=w65, "y-axis"=w64) -> ("MaxPosition"=→"MaxPosition":dbl, "MaxValue"=→"MaxValue":dbl, "MinPosition"=→"MinPosition":dbl, "MinValue"=→"MinValue":dbl)
      }
      frame False {
      }
    }
    n116 = case shown="참" "Save Data" {
      tunnel: w36 -> [w46 w59]
      tunnel: w35 -> [w47 w58]
      tunnel: [w49 w59] -> w38
      tunnel: [w48 w58] -> w37
      frame True {
        n117 = stacked-sequence {
          tunnel: w47 -> [w51]
          tunnel: w46 -> [w52]
          tunnel: [w52] -> w49
          tunnel: [w51] -> w48
          frame #0 {
            n118 = Divide(x=w52, y=sgl 0.15) -> (x/y=w53:sgl[])
            n119 = Build Array (concatenate)(w53, w51) -> (w50:dbl[])
            n120 = call-poly <vilib>:"Write To Spreadsheet File.vi"("transpose? (no:F)"=TRUE ("transpose?\n(no:F)"), "format (%.3f)"="%.6e", "append to file? (new file:F)"=FALSE ("append to file?\n(new file:F)"), "1D data"=w50) -> ()  [unwired: 4 in, 1 out]
          }
        }
      }
      frame False {
      }
    }
    n121 = Unbundle(w28) -> ("System no."=w27:i32, "error out"=w26:errorcluster)
  }
  n122 = call "ERR?.vi"("error in"=w1) -> ("error out"=w4:errorcluster)  [unwired: 17 in, 1 out]
  n123 = call "GCSTranslateError.vi"("error in"=w4) -> ("error out"=w3:errorcluster)  [unwired: 16 in, 2 out]
  n124 = call "Close connection if open.vi"("System no."=w2, "error in"=w3) -> ("error out"=→"error out":errorcluster)  [unwired: 16 in, 1 out]
